vi "OSF Auth Header.vi"(8 "error in":errorcluster, 10 "Token":string="https://api.osf.io/v2/", 11 "client handle":T1) -> (0 "error out":errorcluster, 3 "client handle out":T1)   [LabVIEW 2020]
uses:
  <vilib>/httpClient/ClientHandle.ctl
  <vilib>/httpClient/LabVIEWHTTPClient.lvlib
panel:
  out "resulting string":string
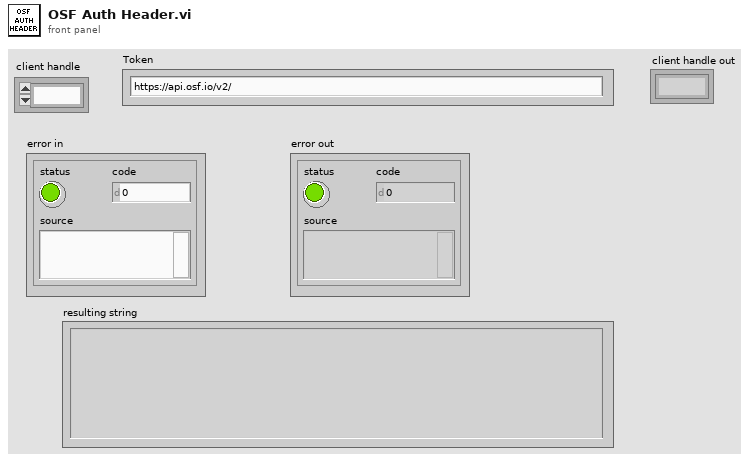
[diagram p1: front panel]
types:
  T1 = typedef "LabVIEWHTTPClient.lvlib/ClientHandle.ctl" = refnum<k1>
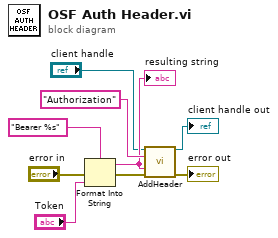
[diagram p0: block diagram]
diagram:
  n1 = Format Into String(format string="Bearer %s", error in="error in", "Token") -> (resulting string=w6:string, error out=w5:errorcluster)  [unwired: 1 in]
  "resulting string" <- w6
  n2 = call <vilib>:"AddHeader.vi"("client handle"="client handle", "header"="Authorization" ("format string"), "value"=w6, "error in (no error)"=w5) -> ("client handle out"=→"client handle out":T1, "error out"=→"error out":errorcluster)  [unwired: 10 in]
